vi "thermocouple graph.vi"() -> ()   [LabVIEW 2025]
uses:
  <vilib>/Utility/file.llb/Write Delimited Spreadsheet (DBL).vi
panel:
  out "Time Stamp":timestamp
  in  "Hold and Clear":bool
  out "Modular Thermalcouple Data":cluster{dbl, dbl}(graph)
  out "Full Thermalcouple Data":cluster{dbl, dbl}(graph)
  in  "?":bool
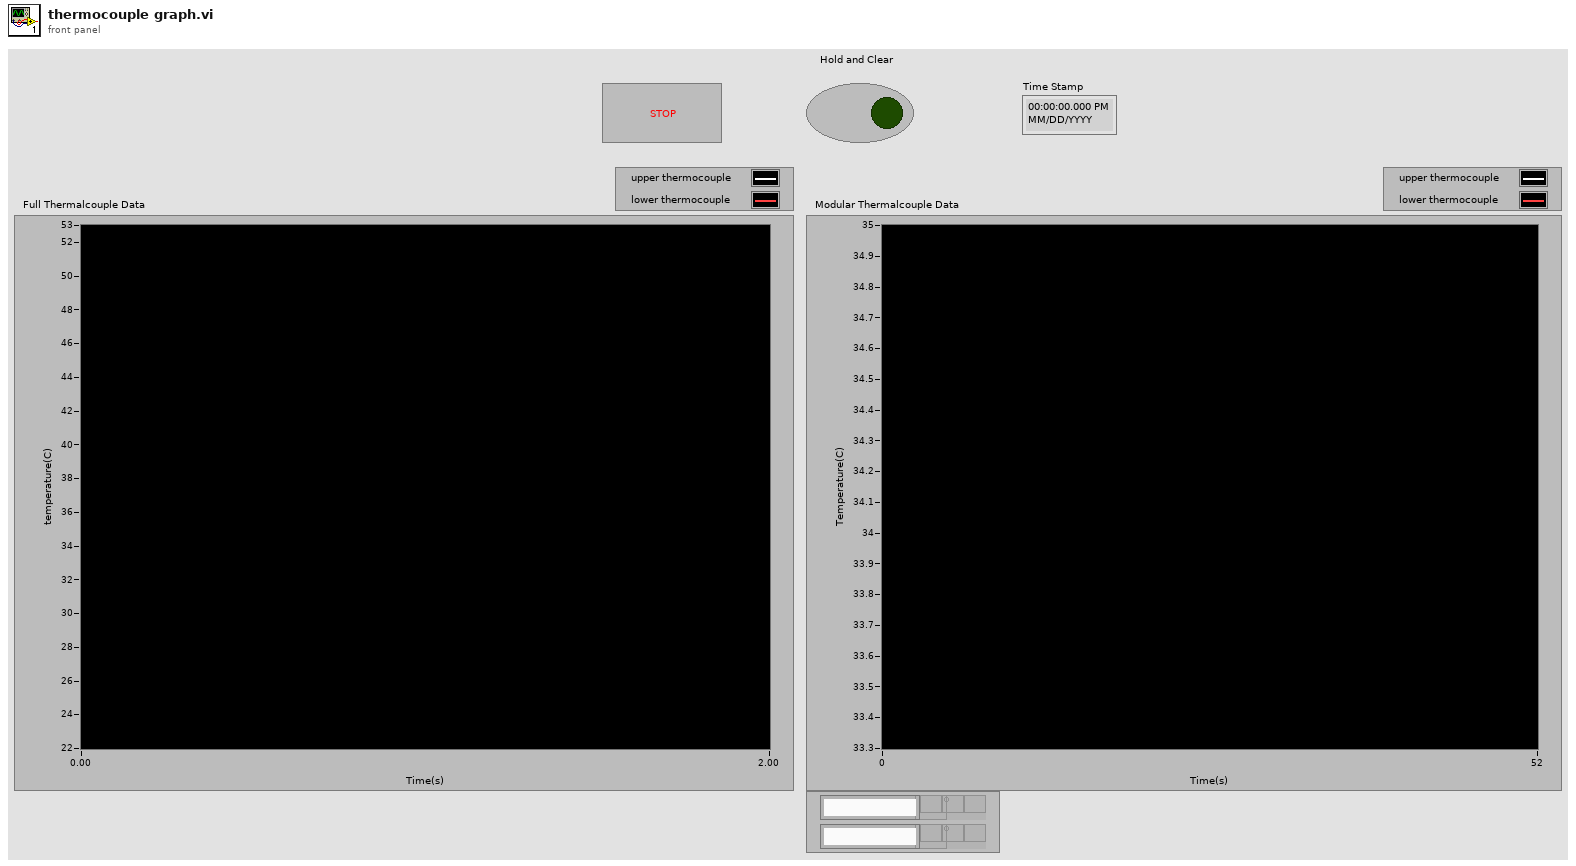
[diagram p1: front panel]
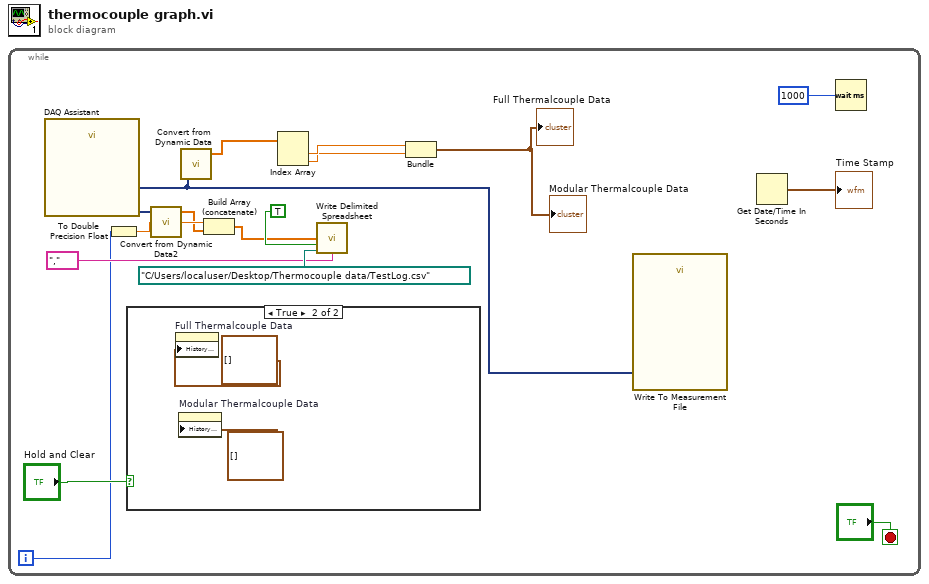
[diagram p0: block diagram]
diagram:
  n1 = while {
    i -> [w4]
    stop <- "?" stop-if-true
    n2 = call "DAQ Assistant"() -> ("data"=w6:dynamicdata)  [unwired: 16 in, 3 out]
    n3 = To Double Precision Float(number=w4) -> (double precision float=w3:dbl)
    n4 = case shown="True" "Hold and Clear" {
      frame False {
      }
      frame True {
        n5 = property on="Full Thermalcouple Data" class="WFChart (strict)"("History Data"=cluster{dbl, dbl}[] []) -> ()  [unwired: 2 in, 2 out]
        n6 = property on="Modular Thermalcouple Data" class="WFChart (strict)"("History Data"=cluster{dbl, dbl}[] []) -> ()  [unwired: 2 in, 2 out]
      }
    }
    n7 = call "Convert from Dynamic Data2"("Dynamic Data Type"=w6) -> ("Array"=w2:dbl[])  [unwired: 3 in]
    n8 = call "Convert from Dynamic Data"("Dynamic Data Type"=w6) -> ("Array"=w16:dbl[])  [unwired: 3 in]
    n9 = Build Array (concatenate)(w3, w2) -> (w1:dbl[])
    n10 = Index Array(array=w16) -> (element #1=w15:dbl, element #2=w14:dbl)  [unwired: 2 in]
    n11 = call-poly <vilib>:"Write Delimited Spreadsheet.vi"("file path (dialog if empty)"=path "C:/Users/localuser/Desktop/Thermocouple data/TestLog.csv", "1D data"=w1, "append to file? (new file:F)"=TRUE, "delimiter (\\t)"="," ("delimiter (\\t)")) -> ()  [unwired: 10 in, 2 out]
    n12 = Bundle(w15, w14) -> (→"Full Thermalcouple Data" →"Modular Thermalcouple Data":cluster{dbl, dbl})  [unwired: 1 in]
    n13 = call "Write To Measurement File"("Signals"=w6) -> ()  [unwired: 16 in, 3 out]
    n14 = Get Date/Time In Seconds() -> (seconds since 1Jan1904=→"Time Stamp":timestamp)
    n15 = Wait (ms)(milliseconds to wait=u32 1000) -> ()  [unwired: 1 out]
  }
